vi "Demo6-Metrics.vi"() -> ()   [LabVIEW 2020]
panel:
  out "Reduced Mean Signal, One Point = One Shot":dbl[](graph)
  in  "IP Address of Remote Device":string="196.254.31.200"
  in  "Disconnect":bool
  out "(For your Reference: )\n Query Sent to Device":string
  # "Diode Demo - Metrics"
  # "Demonstrates simple array queries to the STM32 Diode Device. Does not interpret or plot results."
  # "VI Instructions\n\n1. Make sure you know the Device IP Address.\n2. From Windows command prompt, confirm ping to IP address.\n3. Set up device timings from the Control Panel VI, and then disconnect device from that VI.\n4. Run this VI. (Can only run one VI of the demos at a time.)\n5. When finished exploring queries, disconnect safely from the device via the \"Disconnect\" toggle button. (Not the Abort button).\n\nCreated by Scott Feister on July 18, 2022."
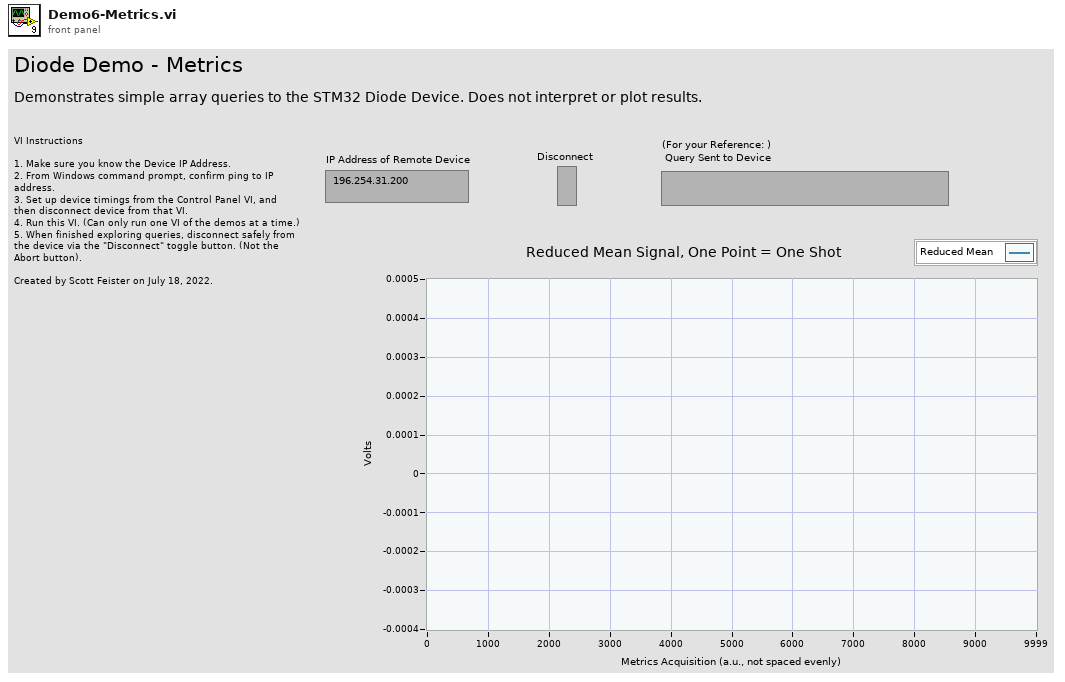
[diagram p1: front panel]
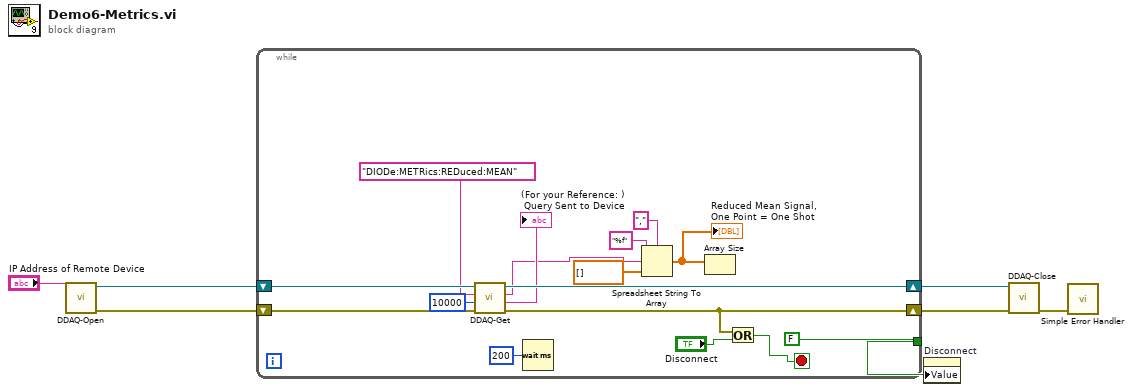
[diagram p0: block diagram]
diagram:
  n1 = call "DDAQ-Open.vi"("IP Address of Nucleo Device"="IP Address of Remote Device") -> ("error out"=w6:errorcluster, "connection ID"=w7:refnum<k5>)  [unwired: 8 in, 1 out]
  n2 = while {
    shift-right: [w21] -> w5
    shift-left: w7 -> [w23]
    shift-right: [w17] -> w4
    shift-left: w6 -> [w22]
    tunnel: [FALSE] -> w2
    stop <- w16 stop-if-true
    n3 = call "DDAQ-Get.vi"("error in (no error)"=w22, "max bytes to read (10000)"=10000 ("max bytes to read (500)"), "SCPI-like Keyword (leave off question mark)"="DIODe:METRics:REDuced:MEAN" ("Diode Keyword (leave off question mark)"), "connection ID"=w23) -> ("error out"=w17:errorcluster, "Query"=→"(For your Reference: )\n Query Sent to Device":string, "Response"=w12:string, "connection ID out"=w21:refnum<k5>)  [unwired: 3 in, 1 out]
    n4 = Wait (ms)(milliseconds to wait=u32 200) -> ()  [unwired: 1 out]
    n5 = Spreadsheet String To Array(delimiter (Tab)=",", format string="%f", spreadsheet string=w12, array type (2D Dbl)=dbl[] []) -> (array=w8:dbl[])
    "Reduced Mean Signal, One Point = One Shot" <- w8
    n6 = Array Size(array=w8) -> ()  [unwired: 1 out]
    n7 = Or(x=w17, y="Disconnect") -> (x .or. y?=w16:bool)
  }
  n8 = property on="Disconnect" class="Bool (strict)"("Value"=w2) -> ()  [unwired: 2 in, 2 out]
  n9 = call "DDAQ-Close.vi"("error in (no error)"=w4, "connection ID"=w5) -> ("error out"=w3:errorcluster)  [unwired: 8 in, 1 out]
  n10 = call <vilib>:"Simple Error Handler.vi"("error in (no error)"=w3) -> ()  [unwired: 4 in, 5 out]
